vi "Timer example.vi"() -> ()   [LabVIEW 2019, in "TimeBenchmark.lvlib"]
uses:
  TimeBenchmark.lvlib
  a34cd281-054a-4b81-a68d-14c84ce3eb44.vi
  80fee96f-9d78-4a77-b50e-07adbf485d80.vi
  3cddb182-5f5a-4b87-8f4f-d469b32a21d6.vi
  b844e3ea-3ce3-42af-a992-45eebbc7281f.vi
  b94a01ef-3d5a-4844-a6c4-475c1b911f1f.vi
  729ad62b-3f87-428c-a42a-403e2d651fbc.vi
  8b285946-094c-4442-8b8c-6dd4a859f54c.vi
  <vilib>/Utility/High Resolution Relative Seconds.vi
  <vilib>/Utility/error.llb/Clear Errors.vi
panel:
  out "elapsed time":dbl
  out "final time":dbl
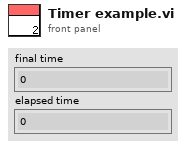
[diagram p1: front panel]
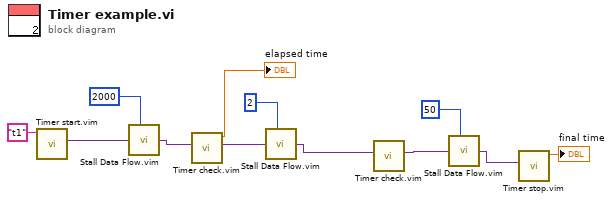
[diagram p0: block diagram]
diagram:
  n1 = call "Timer start.vim"("timer name (t1)"="t1") -> ("dataflow out"=w12:variant)  [unwired: 10 in]
  n2 = call "Stall Data Flow.vim"("value in"=w12, "milliseconds to wait"=u32 2000) -> ("value out"=w8:variant)  [unwired: 1 out]
  n3 = call "Timer check.vim"("dataflow in"=w8) -> ("dataflow out"=w7:variant, "elapsed time"=→"elapsed time":dbl)  [unwired: 9 in]
  n4 = call "Stall Data Flow.vim"("value in"=w7, "milliseconds to wait"=u32 2) -> ("value out"=w6:variant)  [unwired: 1 out]
  n5 = call "Timer check.vim"("dataflow in"=w6) -> ("dataflow out"=w5:variant)  [unwired: 9 in, 1 out]
  n6 = call "Stall Data Flow.vim"("value in"=w5, "milliseconds to wait"=u32 50) -> ("value out"=w4:variant)  [unwired: 1 out]
  n7 = call "Timer stop.vim"("dataflow in"=w4) -> ("final time"=→"final time":dbl)  [unwired: 9 in, 1 out]
